vi "Dequeue.vi"(8 "Error In":errorcluster[](array[cluster]), 11 "QueRef":refnum<queue>) -> (0 "Error Out":errorcluster[](array[cluster]), 1 "Data":variant, 2 "Msg":string, 3 "QueRef":refnum<queue>)   [LabVIEW 2014, in "BusController.lvlib"]
uses:
  BusController.lvlib
  QueueType.ctl
  <vilib>/Utility/error.llb/Error Cluster From Error Code.vi
  <vilib>/ErrorRing/Error Ring.xnode
  <userlib>/NIST/NISTErrorLib/NISTErrorLib.lvlib
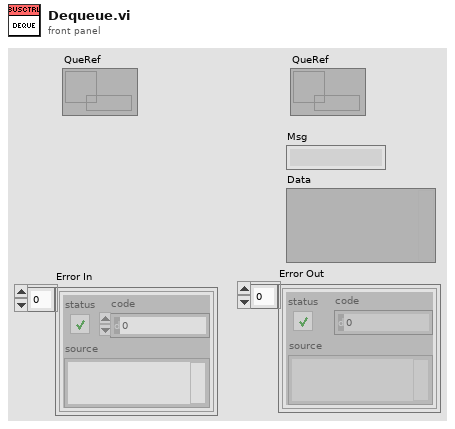
[diagram p1: front panel]
types:
  T1 = typedef "BusController.lvlib/QueueType.ctl" = cluster{"Msg":string, "Data":variant}
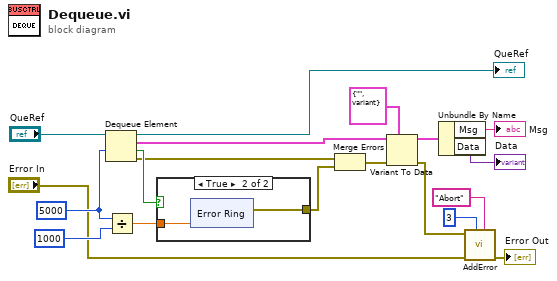
[diagram p0: block diagram]
diagram:
  w19 = 5000 ("timeout in ms (-1)")
  n1 = Dequeue Element(queue="QueRef", timeout in ms (-1)=w19) -> (queue out=→"QueRef":refnum<queue>, element=w12:T1, timed out?=w16:bool, error out=w15:errorcluster)  [unwired: 1 in]
  n2 = Divide(x=w19, y=1000 ("timeout in ms (-1)")) -> (x/y=w17:dbl)
  n3 = case shown="True" w16 {
    tunnel: [_ w21] -> w14
    tunnel: w17 -> [_ w20]
    frame False {
    }
    frame True {
      n4 = xnode "Error Ring"("parameter 0"=w20) -> ("error out"=w21:errorcluster)
    }
  }
  n5 = Merge Errors(w15, w14) -> (w13:errorcluster)
  n6 = Variant To Data(error in=w13, type=T1 {"Msg"="", "Data"=variant} ("QueueType"), Variant=w12) -> (data=w10:T1, error out=w9:errorcluster)
  n7 = Unbundle By Name(w10) -> ("Msg"=→"Msg":string, "Data"=→"Data":variant)
  n8 = call <userlib>:"AddError.vi"("Severity"="Abort", "Priority"=u8 3, "ErrorArray"="Error In", "error in (no error)"=w9) -> ("ErrorArray"=→"Error Out":errorcluster[])  [unwired: 6 in, 1 out]
